vi "Signal config..vi"(11 "base path":path) -> ()   [LabVIEW 2017]
uses:
  <vilib>/Utility/file.llb/Read Delimited Spreadsheet (string).vi
  <vilib>/Utility/file.llb/Write Delimited Spreadsheet (string).vi
panel:
  in  "stop":bool
  in  "Save 3":bool[](array[boolean])
  in  "Save 2":bool[](array[boolean])
  out "Optogenetics related signals":string[](array[string])=["Encoder signal", "Photo-diode", "Distance (cm)", "Photo stimulus signal", "Position in Unity", "Valve open", "Lick signal", "Frame signal", "Stimulus protocol", "VR context", "Analog lick signal", "EyeCam frame signal", "Masking light signal", "Frame signal 2"]
  out "Behavior and task related signals":string[](array[string])=["Encoder signal", "Photo-diode", "Distance (cm)", "Photo stimulus signal", "Position in Unity", "Valve open", "Lick signal", "Frame signal", "Stimulus protocol", "VR context", "Analog lick signal", "EyeCam frame signal", "Masking light signal", "Frame signal 2"]
  in  "Save":bool[](array[boolean])
  out "Imaging ralated signals":string[](array[string])=["Encoder signal", "Photo-diode", "Distance (cm)", "Photo stimulus signal", "Position in Unity", "Valve open", "Lick signal", "Frame signal", "Stimulus protocol", "VR context", "Analog lick signal", "EyeCam frame signal", "Masking light signal", "Frame signal 2"]
  # "P0.5"
  # "Dev1/ctr0"
  # "P0.3"
  # "AI 4"
  # "AI 1"
  # "Calculated in LV"
  # "AI 3"
  # "Feedback from Unity"
  # "P0.6"
  # "P0.4"
  # "AI 0"
  # "AI 6"
  # "AI 2"
  # "LV command"
  # "LV command"
  # "LV command"
  # "AI 5"
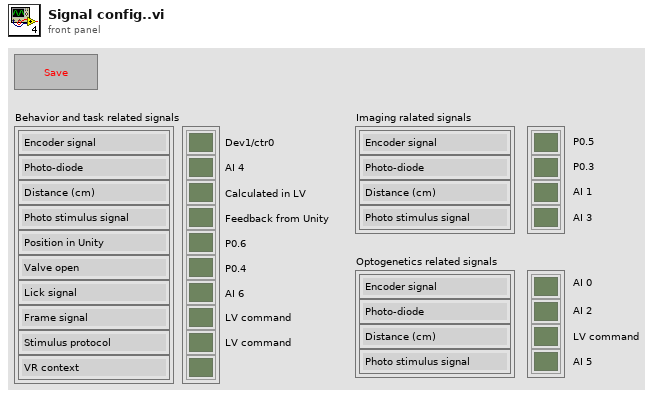
[diagram p1: front panel]
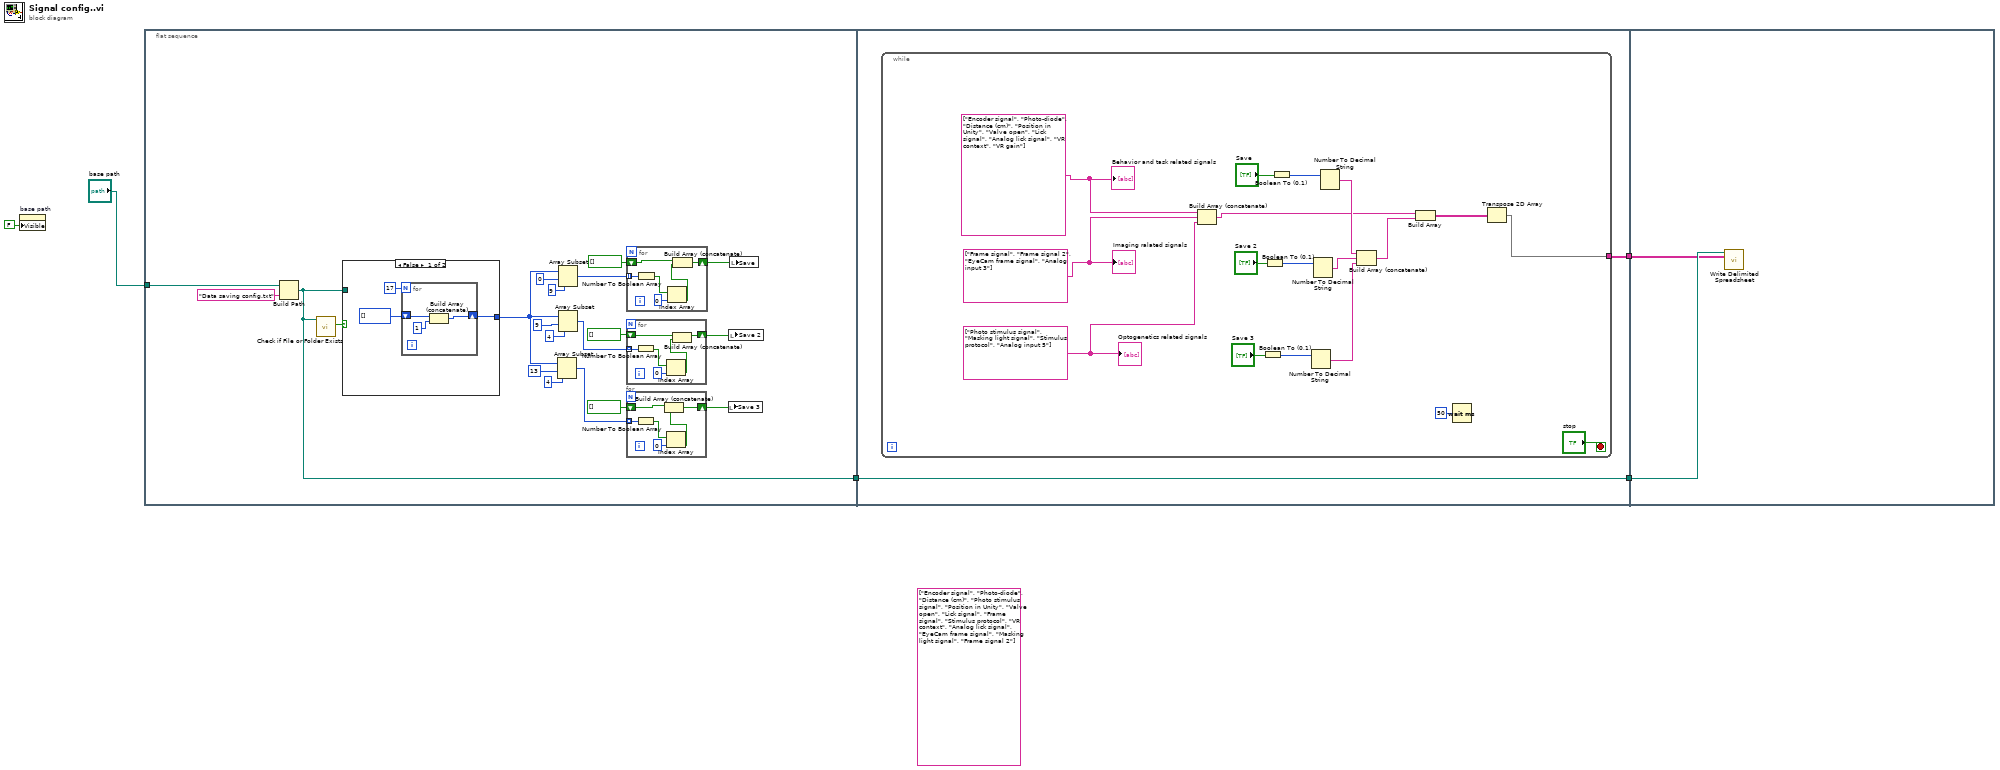
[diagram p0: block diagram]
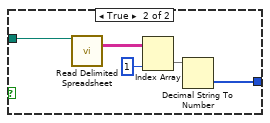
[diagram p2: hidden frame]
diagram:
  (unwired) string[] ["Encoder signal", "Photo-diode", "Distance (cm)", "Photo stimulus signal", "Position in Unity", "Valve open", "Lick signal", "Frame signal", "Stimulus protocol", "VR context", "Analog lick signal", "EyeCam frame signal", "Masking light signal", "Frame signal 2"] ("channel name(s) in (Untitled)")
  n1 = property on="base path" class="Path"("Visible"=FALSE) -> ()  [unwired: 2 in, 2 out]
  n2 = flat-sequence {
    tunnel: [w8] -> w5
    tunnel: "base path" -> [w6]
    tunnel: w5 -> [w56]
    tunnel: [w56] -> w4
    tunnel: [w55] -> w3
    tunnel: w4 -> [w76]
    tunnel: w3 -> [w75]
    frame #0 {
      n3 = Build Path(base path=w6, name or relative path="Data saving config.txt") -> (appended path=w8:path)
      n4 = call <vilib>:"Check if File or Folder Exists.vi"("path"=w8) -> ("file or folder exists?"=w7:bool)  [unwired: 8 in, 2 out]
      n5 = case shown="False" w7 {
        tunnel: [w28 w33] -> w18
        tunnel: w8 -> [_ w32]
        frame False {
          n6 = for {
            N: 17 -> [_]
            shift-right: [w30] -> w28
            shift-left: i32[] [] -> [w31]
            n7 = Build Array (concatenate)(w31, 1 ("index")) -> (w30:i32[])
          }
        }
        frame True {
          n8 = call-poly <vilib>:"Read Delimited Spreadsheet.vi"("file path (dialog if empty)"=w32) -> ("all rows"=w36:string[][])  [unwired: 9 in, 5 out]
          n9 = Index Array(array=w36, index (col)=1 ("disabled index (col)")) -> (element=w34:string[])  [unwired: 1 in]
          n10 = Decimal String To Number(string=w34) -> (number=w33:i32[])  [unwired: 2 in, 1 out]
        }
      }
      n11 = Array Subset(array=w18, index=13, length=4) -> (w11:i32[])
      n12 = Array Subset(array=w18, index=0, length=9) -> (w17:i32[])
      n13 = Array Subset(array=w18, index=9, length=4) -> (w12:i32[])
      n14 = for {
        tunnel: w12 -> [w48] mode=indexing
        shift-right: [w44] -> w10
        shift-left: bool[] [] -> [w43]
        n15 = Number To Boolean Array(number=w48) -> (Boolean array=w46:bool[])
        n16 = Index Array(array=w46, index=0) -> (element=w47:bool)
        n17 = Build Array (concatenate)(w43, w47) -> (w44:bool[])
      }
      n18 = for {
        tunnel: w11 -> [w42] mode=indexing
        shift-right: [w38] -> w9
        shift-left: bool[] [] -> [w37]
        n19 = Number To Boolean Array(number=w42) -> (Boolean array=w40:bool[])
        n20 = Index Array(array=w40, index=0) -> (element=w41:bool)
        n21 = Build Array (concatenate)(w37, w41) -> (w38:bool[])
      }
      n22 = for {
        tunnel: w17 -> [w54] mode=indexing
        shift-right: [w50] -> w15
        shift-left: bool[] [] -> [w49]
        n23 = Number To Boolean Array(number=w54) -> (Boolean array=w52:bool[])
        n24 = Index Array(array=w52, index=0) -> (element=w53:bool)
        n25 = Build Array (concatenate)(w49, w53) -> (w50:bool[])
      }
      n26 = local write "Save 3"(w9) -> ()
      n27 = local write "Save 2"(w10) -> ()
      n28 = local write "Save"(w15) -> ()
    }
    frame #1 {
      n29 = while {
        tunnel: [w59] -> w55
        stop <- "stop" stop-if-true
        w63 = string[] ["Photo stimulus signal", "Masking light signal", "Stimulus protocol", "Analog input 5"] ("channel name(s) in (Untitled)")
        w64 = string[] ["Frame signal", "Frame signal 2", "EyeCam frame signal", "Analog input 3"] ("channel name(s) in (Untitled)")
        w65 = string[] ["Encoder signal", "Photo-diode", "Distance (cm)", "Position in Unity", "Valve open", "Lick signal", "Analog lick signal", "VR context", "VR gain"] ("channel name(s) in (Untitled)")
        n30 = Build Array (concatenate)(w65, w64, w63) -> (w62:string[])
        n31 = Boolean To (0,1)(Boolean="Save 3") -> (0, 1=w70:i16[])
        n32 = Boolean To (0,1)(Boolean="Save 2") -> (0, 1=w72:i16[])
        n33 = Boolean To (0,1)(Boolean="Save") -> (0, 1=w73:i16[])
        n34 = Number To Decimal String(number=w70) -> (decimal integer string=w67:string[])  [unwired: 1 in]
        n35 = Number To Decimal String(number=w72) -> (decimal integer string=w68:string[])  [unwired: 1 in]
        n36 = Number To Decimal String(number=w73) -> (decimal integer string=w66:string[])  [unwired: 1 in]
        n37 = Build Array (concatenate)(w66, w68, w67) -> (w61:string[])
        n38 = Build Array(w62, w61) -> (w60:string[][])
        n39 = Wait (ms)(milliseconds to wait=u32 50) -> ()  [unwired: 1 out]
        n40 = Transpose 2D Array(2D array=w60) -> (transposed array=w59:string[][])
        "Imaging ralated signals" <- w64
        "Behavior and task related signals" <- w65
        "Optogenetics related signals" <- w63
      }
    }
    frame #2 {
      n41 = call-poly <vilib>:"Write Delimited Spreadsheet.vi"("file path (dialog if empty)"=w76, "2D data"=w75) -> ()  [unwired: 12 in, 2 out]
    }
  }
